vi "Keysight XSAnVMA-Example1.vi"() -> ()   [LabVIEW 2021, in "Keysight XSAnVMA.lvlib"]
doc: "Initializes the driver, reads a few Identity interface properties, and checks the instrument error queue. May include additional instrument specific functionality."
uses:
  <instrlib>/Keysight XSAnVMA/Keysight XSAnVMA.lvlib
  Keysight XSAn/Keysight XSAn.lvlib
panel:
  in  "AttributeValue":dbl=2610000000.0
  in  "DigitalDemodTrace":string="AverageMode"
  out "ValActualSize":i32
  out "Waveform Output":dbl[](array[numeric]) format="%.2p"
  in  "MaxTime":i32=20000 caption="MaxTime (ms)"
  in  "PersonalityName":string="VMA"
  out "Simulation":bool
  out "Identity Properties":string[](array[string])
  out "MESSAGE BOX":string
  in  "option string":string="DriverSetup= Model=, Trace=false, TraceName=c:\\\\temp\\\\traceOut"
  in  "select":bool=TRUE
  in  "Resource string":string="TCPIP0::146.208.245.241::hislip0::INSTR" caption="resource string"
  in  "Simulate":bool=TRUE
  # "Keysight XSAnVMA - Example 1"
  # "SYSTEM_DRIVER_PREFIX"
  # ":"
  # ":"
  # "SYSTEM_DRIVER_REVISION"
  # "SYSTEM_DRIVER_VENDOR"
  # ":"
  # "SPECIFIC_DRIVER_DESCRIPTION"
  # ":"
  # "INSTRUMNET_MODEL"
  # ":"
  # "INSTRUMENT_FIRMWARE_REVISION"
  # ":"
  # "SIMULATE"
  # ":"
  # "© Keysight Technologies 2018 - 2019"
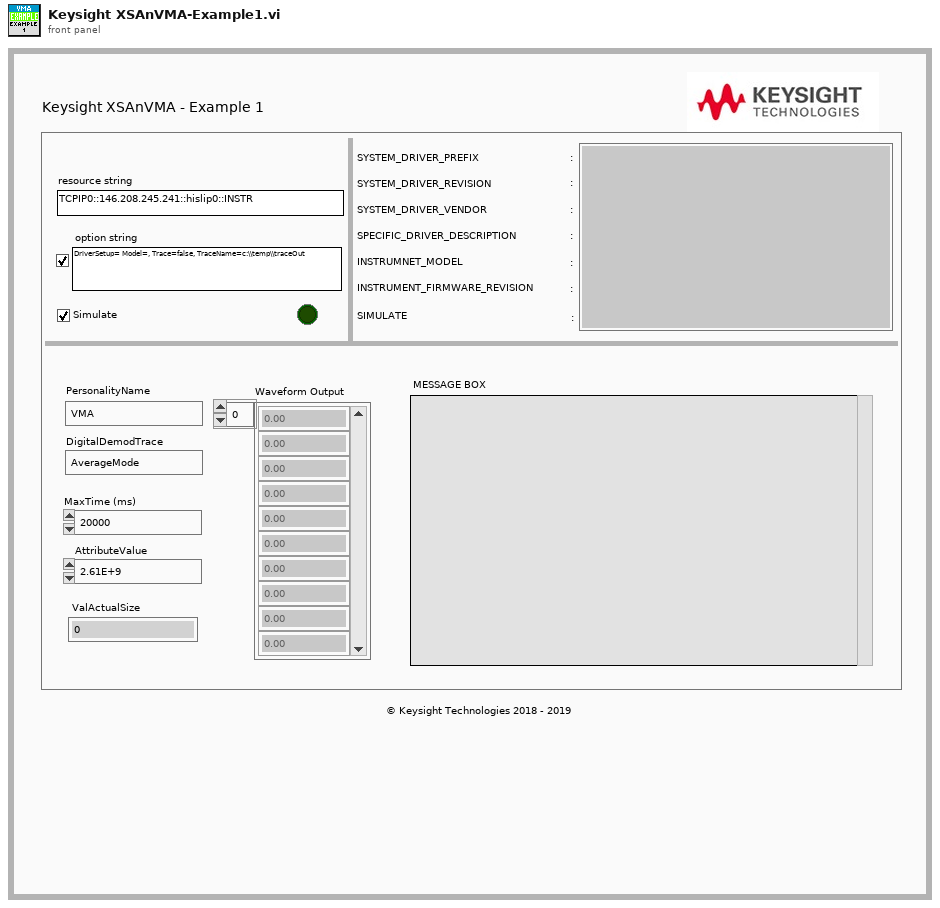
[diagram p1: front panel]
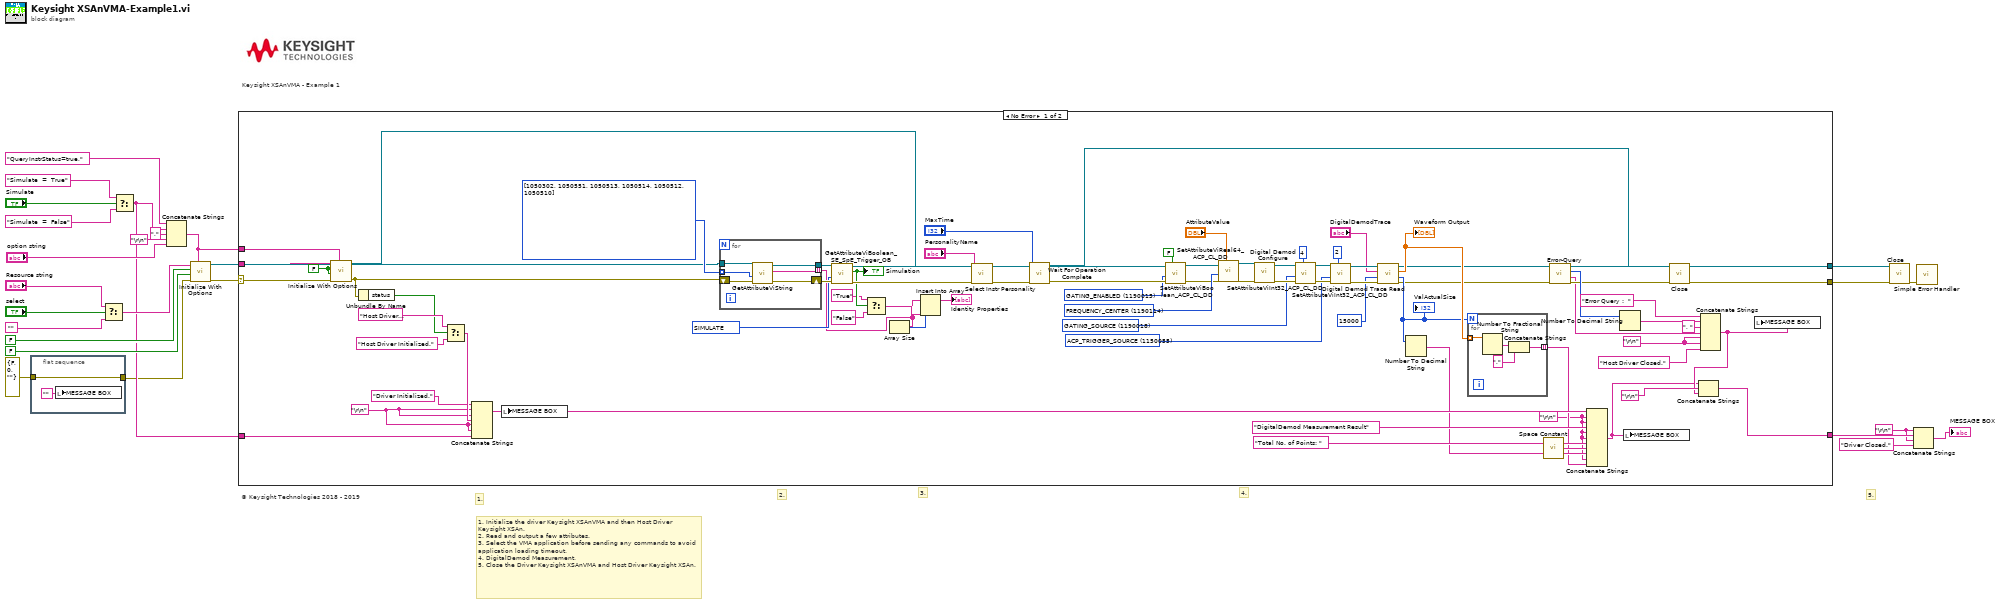
[diagram p0: block diagram]
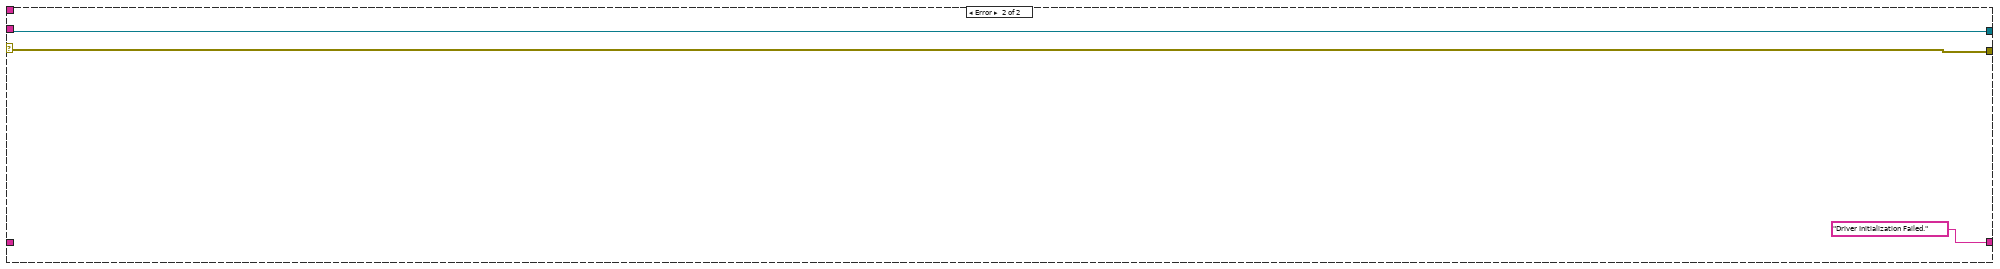
[diagram p2: hidden frame]
diagram:
  w2 = "\r\n"
  # "5."
  # "4."
  # "© Keysight Technologies 2018 - 2019"
  # "3."
  # "2."
  # "Keysight XSAnVMA - Example 1"
  # "1."
  # "1. Initialize the driver Keysight XSAnVMA and then Host Driver Keysight XSAn. \n2. Read and output a few attributes.\n3. Select the VMA application before sending any commands to avoid application loading timeout.\n4. DigitalDemod Measurement.\n5. Close the Driver Keysight XSAnVMA and Host Driver Keysight XSAn."
  n1 = flat-sequence {
    tunnel: errorcluster {"status"=FALSE, "code"=0, "source"=""} ("error in (no error)") -> [w27]
    tunnel: [w27] -> w9
    frame #0 {
      n2 = local write "MESSAGE BOX"("") -> ()
    }
  }
  n3 = Select(t="Resource string", s="select", f="") -> (s? t:f=w12:string)
  n4 = Select(t="Simulate  =  True", s="Simulate", f="Simulate  =  False" ("t")) -> (s? t:f=w11:string)
  n5 = Concatenate Strings("QueryInstrStatus=true," ("t"), w11, "," ("string"), "\r\n", "option string") -> (w13:string)
  n6 = call "Initialize With Options.vi"("option string"=w13, "error in (no error)"=w9, "reset device (Off)"=FALSE ("id query (Off)"), "id query (Off)"=FALSE, "resource string"=w12) -> ("error out"=w3:errorcluster, "instrument handle out"=w14:refnum<k15>)  [unwired: 5 in]
  n7 = case shown="No Error" w3 {
    selector: w3 -> [w41 w119]
    tunnel: w14 -> [w72 w118]
    tunnel: w13 -> [w68 _]
    tunnel: w12 -> [w67 _]
    tunnel: w11 -> [w63 _]
    tunnel: [w36 w119] -> w7
    tunnel: [w43 w118] -> w6
    tunnel: [w33 "Driver Initialization Failed." ("string")] -> w5
    frame No Error {
      w35 = "\r\n"
      w47 = "\r\n"
      w69 = FALSE ("id query (Off)")
      w83 = u32 1150055 items=["ACP_AVERAGE_COUNT"=1150010, "ACP_AVERAGE_MODE"=1150012, "ACP_CARRIER_COUNT"=1150013, "ACP_CARRIER_POWER_REFERENCE_TYPE"=1191309, "ACP_CARRIER_REFERENCE_NUMBER"=1150019, "ACP_DETECTOR_TYPE"=1150003, "ACP_DISPLAY_VIEW_SELECTION"=1191352, "ACP_DISPLAY_WINDOWY_REF_POSITION"=1190656, "ACP_FAST_POWER_IF_GAIN"=1191705, "ACP_FAST_POWER_RBW_MODE"=1191704, "ACP_FREQUENCY_PHASE_NOISE_OPTION_STATE"=1150081, "ACP_MARKER_ACTIVE_MARKER"=1150095, "ACP_MARKER_DELTA_REFERENCE"=1150099, "ACP_MARKER_TRACE"=1150040, "ACP_MARKER_TYPE"=1150102, "ACP_MEASUREMENT_METHOD"=1150006, "ACP_MEASUREMENT_TYPE"=1150007, "ACP_POWER_SPECTRAL_DENSITY_REFERENCE"=1150009, "ACP_SWEEPCOUPLING_BANDWIDTH_SHAPE"=1150001, "ACP_SWEEPCOUPLING_BANDWIDTH_TYPE"=1150002, "ACP_SWEEPCOUPLING_SWEEP_POINTS"=1150025, "ACP_SWEEPCOUPLING_SWEEP_TIME_AUTO_RULES"=1150029, "ACP_TRIGGER_SOURCE"=1150055, "ANALOG_ANTI_ALIASING_FILTER_TYPE"=1191706, "DIGITAL_DEMOD_AVERAGE_COUNT"=1191759, "DIGITAL_DEMOD_AVERAGE_MODE"=1191757, "DIGITAL_DEMOD_CPM_INDEX"=1191642, "DIGITAL_DEMOD_DISPLAY_BITS_FORMAT"=1191625, "DIGITAL_DEMOD_DISPLAY_IDEAL_STATE_SHAPE"=1191615, "DIGITAL_DEMOD_DISPLAY_VIEW_SELECTION"=1191588, "DIGITAL_DEMOD_DISPLAY_WINDOW_TRACE_DATA_FORMAT"=1191665, "DIGITAL_DEMOD_DISPLAY_WINDOW_TRACE_DATA_TYPE"=1191666, "DIGITAL_DEMOD_DISPLAY_WINDOW_X_REF_POSITION"=1191610, "DIGITAL_DEMOD_DISPLAY_WINDOW_X_TIME_UNIT"=1191614, "DIGITAL_DEMOD_DISPLAY_WINDOW_Y_POSITION"=1191592, "DIGITAL_DEMOD_EQUALIZATION_FILTER_LENGTH"=1191634, "DIGITAL_DEMOD_EVM_NORMALIZATION_REFERENCE"=1191667, "DIGITAL_DEMOD_FILTER_REFERENCE"=1191630, "DIGITAL_DEMOD_FILTER_TYPE"=1191627, "DIGITAL_DEMOD_LIMITS_CLOCK_ERROR_UNIT"=1191620, "DIGITAL_DEMOD_LIMITS_FREQUENCY_ERROR_UNIT"=1191621, "DIGITAL_DEMOD_MARKER_ACTIVE_MARKER"=1191593, "DIGITAL_DEMOD_MARKER_DELTA_REFERENCE"=1191596, "DIGITAL_DEMOD_MARKER_FUNCTION"=1191607, "DIGITAL_DEMOD_MARKER_TYPE"=1191601, "DIGITAL_DEMOD_MODULATION_FORMAT"=1191637, "DIGITAL_DEMOD_PHASE_NOISE_OPTIMIZATION"=1191660, "DIGITAL_DEMOD_POINTS_PER_SAMPLE"=1191626, "DIGITAL_DEMOD_SYNC_OFFSET"=1191650, "DIGITAL_DEMOD_TRACE_LIMIT_TYPE"=1191676, "DIGITAL_DEMOD_TRACE_LIMIT_WINDOW_LIMIT"=1191678, "DIGITAL_DEMOD_TRACE_LIMIT_X_REFERENCE"=1191677, "DIGITAL_DEMOD_TRACE_LIMIT_X_UNIT"=1191672, "DIGITAL_DEMOD_TRACE_LIMIT_Y_UNIT"=1191761, "DIGITAL_DEMOD_TRIGGER_SOURCE"=1191613, "GATING_DELAY_COMPENSATION"=1150141, "GATING_SOURCE"=1190018, "GATING_TYPE"=1190019, "INPUT_IQ_FEED_TYPE"=1190844, "INPUT_IQ_I_COUPLING"=1191695, "INPUT_IQ_I_IMPEDANCE"=1191701, "INPUT_IQ_IMPEDANCE"=1191699, "INPUT_IQ_Q_COUPLING"=1191696, "INPUT_IQ_Q_IMPEDANCE"=1191702, "INPUT_RF_PRE_AMPLIFIER_BAND"=1190118, "LEVEL_ATTENUATION_OPTIMIZE"=1190119, "LEVEL_ATTENUATION_STEP_INCREMENT"=1190120] ("AttributeID")
      w87 = u32 1190018 items=["ACP_AVERAGE_COUNT"=1150010, "ACP_AVERAGE_MODE"=1150012, "ACP_CARRIER_COUNT"=1150013, "ACP_CARRIER_POWER_REFERENCE_TYPE"=1191309, "ACP_CARRIER_REFERENCE_NUMBER"=1150019, "ACP_DETECTOR_TYPE"=1150003, "ACP_DISPLAY_VIEW_SELECTION"=1191352, "ACP_DISPLAY_WINDOWY_REF_POSITION"=1190656, "ACP_FAST_POWER_IF_GAIN"=1191705, "ACP_FAST_POWER_RBW_MODE"=1191704, "ACP_FREQUENCY_PHASE_NOISE_OPTION_STATE"=1150081, "ACP_MARKER_ACTIVE_MARKER"=1150095, "ACP_MARKER_DELTA_REFERENCE"=1150099, "ACP_MARKER_TRACE"=1150040, "ACP_MARKER_TYPE"=1150102, "ACP_MEASUREMENT_METHOD"=1150006, "ACP_MEASUREMENT_TYPE"=1150007, "ACP_POWER_SPECTRAL_DENSITY_REFERENCE"=1150009, "ACP_SWEEPCOUPLING_BANDWIDTH_SHAPE"=1150001, "ACP_SWEEPCOUPLING_BANDWIDTH_TYPE"=1150002, "ACP_SWEEPCOUPLING_SWEEP_POINTS"=1150025, "ACP_SWEEPCOUPLING_SWEEP_TIME_AUTO_RULES"=1150029, "ACP_TRIGGER_SOURCE"=1150055, "ANALOG_ANTI_ALIASING_FILTER_TYPE"=1191706, "DIGITAL_DEMOD_AVERAGE_COUNT"=1191759, "DIGITAL_DEMOD_AVERAGE_MODE"=1191757, "DIGITAL_DEMOD_CPM_INDEX"=1191642, "DIGITAL_DEMOD_DISPLAY_BITS_FORMAT"=1191625, "DIGITAL_DEMOD_DISPLAY_IDEAL_STATE_SHAPE"=1191615, "DIGITAL_DEMOD_DISPLAY_VIEW_SELECTION"=1191588, "DIGITAL_DEMOD_DISPLAY_WINDOW_TRACE_DATA_FORMAT"=1191665, "DIGITAL_DEMOD_DISPLAY_WINDOW_TRACE_DATA_TYPE"=1191666, "DIGITAL_DEMOD_DISPLAY_WINDOW_X_REF_POSITION"=1191610, "DIGITAL_DEMOD_DISPLAY_WINDOW_X_TIME_UNIT"=1191614, "DIGITAL_DEMOD_DISPLAY_WINDOW_Y_POSITION"=1191592, "DIGITAL_DEMOD_EQUALIZATION_FILTER_LENGTH"=1191634, "DIGITAL_DEMOD_EVM_NORMALIZATION_REFERENCE"=1191667, "DIGITAL_DEMOD_FILTER_REFERENCE"=1191630, "DIGITAL_DEMOD_FILTER_TYPE"=1191627, "DIGITAL_DEMOD_LIMITS_CLOCK_ERROR_UNIT"=1191620, "DIGITAL_DEMOD_LIMITS_FREQUENCY_ERROR_UNIT"=1191621, "DIGITAL_DEMOD_MARKER_ACTIVE_MARKER"=1191593, "DIGITAL_DEMOD_MARKER_DELTA_REFERENCE"=1191596, "DIGITAL_DEMOD_MARKER_FUNCTION"=1191607, "DIGITAL_DEMOD_MARKER_TYPE"=1191601, "DIGITAL_DEMOD_MODULATION_FORMAT"=1191637, "DIGITAL_DEMOD_PHASE_NOISE_OPTIMIZATION"=1191660, "DIGITAL_DEMOD_POINTS_PER_SAMPLE"=1191626, "DIGITAL_DEMOD_SYNC_OFFSET"=1191650, "DIGITAL_DEMOD_TRACE_LIMIT_TYPE"=1191676, "DIGITAL_DEMOD_TRACE_LIMIT_WINDOW_LIMIT"=1191678, "DIGITAL_DEMOD_TRACE_LIMIT_X_REFERENCE"=1191677, "DIGITAL_DEMOD_TRACE_LIMIT_X_UNIT"=1191672, "DIGITAL_DEMOD_TRACE_LIMIT_Y_UNIT"=1191761, "DIGITAL_DEMOD_TRIGGER_SOURCE"=1191613, "GATING_DELAY_COMPENSATION"=1150141, "GATING_SOURCE"=1190018, "GATING_TYPE"=1190019, "INPUT_IQ_FEED_TYPE"=1190844, "INPUT_IQ_I_COUPLING"=1191695, "INPUT_IQ_I_IMPEDANCE"=1191701, "INPUT_IQ_IMPEDANCE"=1191699, "INPUT_IQ_Q_COUPLING"=1191696, "INPUT_IQ_Q_IMPEDANCE"=1191702, "INPUT_RF_PRE_AMPLIFIER_BAND"=1190118, "LEVEL_ATTENUATION_OPTIMIZE"=1190119, "LEVEL_ATTENUATION_STEP_INCREMENT"=1190120] ("AttributeID")
      w94 = u32 1190114 items=["ACP_CARRIER_CPSD"=1150014, "ACP_CARRIER_REFERENCE_FREQUENCY"=1150015, "ACP_CARRIER_REFERENCE_LEVEL"=1150017, "ACP_DISPLAY_WINDOWY_REFERENCE"=1150091, "ACP_DISPLAY_WINDOWY_SCALE"=1150092, "ACP_FREQUENCY_SPAN"=1150094, "ACP_INTEGRATION_BANDWIDTH"=1191694, "ACP_MARKER_POSITION"=1150101, "ACP_MARKER_TRACE_POINTS_POSITION"=1190657, "ACP_OFFSET_FILTER_ALPHA"=1150103, "ACP_SWEEPCOUPLING_RESOLUTION_BANDWIDTH"=1150023, "ACP_SWEEPCOUPLING_SWEEP_TIME"=1150027, "ACP_SWEEPCOUPLING_VIDEO_BANDWIDTH"=1150030, "DIGITAL_DEMOD_ADJUST_CLOCK"=1191641, "DIGITAL_DEMOD_APSK_RING2_RATIO"=1191631, "DIGITAL_DEMOD_APSK_RING3_RATIO"=1191632, "DIGITAL_DEMOD_DISPLAY_IDEAL_STATE_SIZE"=1191616, "DIGITAL_DEMOD_DISPLAY_WINDOW_X_REFERENCE"=1191609, "DIGITAL_DEMOD_DISPLAY_WINDOW_X_WIDTH"=1191658, "DIGITAL_DEMOD_DISPLAY_WINDOW_Y_REFERENCE"=1191591, "DIGITAL_DEMOD_DISPLAY_WINDOW_Y_SCALE"=1191590, "DIGITAL_DEMOD_EQUALIZATION_CONVERGENCE"=1191636, "DIGITAL_DEMOD_FILTER_ALPHA"=1191628, "DIGITAL_DEMOD_FILTER_BETA"=1191629, "DIGITAL_DEMOD_FSK_DEVIATION_REFERENCE"=1191638, "DIGITAL_DEMOD_FSK_TX_FREQUENCY_OFFSET"=1191640, "DIGITAL_DEMOD_IQ_ROTATION"=1191664, "DIGITAL_DEMOD_LIMITS_CLOCK_ERROR_IN_HERTZ"=1191619, "DIGITAL_DEMOD_LIMITS_CLOCK_ERROR_INPPM"=1191622, "DIGITAL_DEMOD_LIMITS_DEVIATION_ACCURACY"=1191647, "DIGITAL_DEMOD_LIMITS_FREQUENCY_ERROR_IN_HERTZ"=1191618, "DIGITAL_DEMOD_LIMITS_FREQUENCY_ERROR_INPPM"=1191623, "DIGITAL_DEMOD_LIMITS_POWER_LIMIT"=1191624, "DIGITAL_DEMOD_LIMITS_RMS_FSK_ERROR"=1191646, "DIGITAL_DEMOD_LIMITS_RMS_OFFSETEVM"=1191648, "DIGITAL_DEMOD_MARKER_FUNCTION_BAND_LEFT"=1191602, "DIGITAL_DEMOD_MARKER_FUNCTION_BAND_RIGHT"=1191603, "DIGITAL_DEMOD_MARKER_FUNCTION_BAND_SPAN"=1191604, "DIGITAL_DEMOD_MARKER_POSITION"=1191599, "DIGITAL_DEMOD_MARKER_WINDOW_TRACE"=1191681, "DIGITAL_DEMOD_MARKER_Y_IMAGINARY"=1191682, "DIGITAL_DEMOD_MULTI_CARRIER_FILTER_BANDWIDTH"=1191680, "DIGITAL_DEMOD_SAMPLE_RATE"=1191617, "DIGITAL_DEMOD_SWEEP_COUPLING_RESOLUTION_BANDWIDTH"=1191762, "DIGITAL_DEMOD_SYMBOL_INTERVAL"=1191659, "DIGITAL_DEMOD_SYNC_BURST_SEARCH_THRESHOLD"=1191652, "DIGITAL_DEMOD_SYNC_SEARCH_LENGTH"=1191653, "DIGITAL_DEMOD_TRACE_LIMIT_MARGIN"=1191674, "DIGITAL_DEMOD_TRACE_LIMIT_X_OFFSET"=1191673, "DIGITAL_DEMOD_TRACE_LIMIT_Y_OFFSET"=1191760, "FREQUENCY_CENTER"=1190114, "FREQUENCY_CENTER_STEP"=1150133, "GATING_DELAY"=1190014, "GATING_HOLD_OFF_TIME"=1150142, "GATING_LENGTH"=1190016, "GATING_VIEW_START_TIME"=1191460, "GATING_VIEW_SWEEP_TIME"=1190021, "INPUT_IQ_CENTER_FREQUENCY"=1191715, "INPUT_IQ_I_ATTENUATION"=1190851, "INPUT_IQ_I_ATTENUATION_RATIO"=1190853, "INPUT_IQ_I_EXTERNAL_GAIN"=1190840, "INPUT_IQ_I_OFFSET"=1191697, "INPUT_IQ_I_SKEW_FACTOR"=1190843, "INPUT_IQ_Q_ATTENUATION_RATIO"=1190854, "INPUT_IQ_Q_ATTENUATION"=1190852, "INPUT_IQ_Q_EXTERNAL_GAIN"=1190841, "INPUT_IQ_Q_OFFSET"=1191698, "INPUT_IQ_Q_SKEW_FACTOR"=1190842, "INPUT_IQ_REFERENCE_IMPEDANCE"=1191700, "INPUT_RF_BASE_STATION_GAIN"=1190115, "INPUT_RF_MOBILE_STATION_GAIN"=1190116, "LEVEL_ATTENUATION"=1190002, "LEVEL_ELECTRONIC_ATTENUATION"=1190121] ("AttributeID")
      w96 = u32 1190015 items=["ACP_AVERAGE_ENABLED"=1150011, "ACP_CARRIER_REFERENCE_FREQUENCY_AUTO_ENABLED"=1150016, "ACP_CARRIER_REFERENCE_LEVEL_AUTO_ENABLED"=1150018, "ACP_CARRIER_REFERENCE_NUMBER_AUTO_ENABLED"=1150020, "ACP_DETECTOR_AUTO_ENABLED"=1150058, "ACP_DISPLAY_BAR_GRAPH_ENABLED"=1150089, "ACP_DISPLAY_WINDOWY_AUTO_SCALE_ENABLED"=1150093, "ACP_FREQUENCY_PHASE_NOISE_OPTION_AUTO_ENABLED"=1150072, "ACP_LIMIT_TEST_ENABLED"=1150005, "ACP_LIMIT_TEST_FAIL_STATE"=1150004, "ACP_MARKER_COUPLE_ENABLED"=1150098, "ACP_MARKER_ENABLED"=1150100, "ACP_NOISE_CORRECTION_ENABLED"=1150008, "ACP_OFFSET_FILTER_ENABLED"=1150104, "ACP_SWEEPCOUPLING_RESOLUTION_BANDWIDTH_AUTO_ENABLED"=1150024, "ACP_SWEEPCOUPLING_SWEEP_TIME_AUTO_ENABLED"=1150028, "ACP_SWEEPCOUPLING_VIDEO_BANDWIDTH_AUTO_ENABLED"=1150033, "ANALOG_ANTI_ALIASING_FILTER_AUTO_ENABLED"=1191707, "AUTO_SCALE_ENABLED"=1191693, "CONTINUOUS_PEAK_SEARCH_ENABLED"=1191709, "DIGITAL_DEMOD_AVERAGE_ENABLED"=1191758, "DIGITAL_DEMOD_CPM_AUTO_ENABLED"=1191643, "DIGITAL_DEMOD_DISPLAY_WINDOW_X_AUTO_SCALE_ENABLED"=1191608, "DIGITAL_DEMOD_EQUALIZATION_ENABLED"=1191633, "DIGITAL_DEMOD_EQUALIZATION_HOLD_ENABLED"=1191635, "DIGITAL_DEMOD_FSK_DEVIATION_REFERENCE_AUTO_ENABLED"=1191639, "DIGITAL_DEMOD_IF_GAIN"=1191656, "DIGITAL_DEMOD_IF_GAIN_AUTO_ENABLED"=1191657, "DIGITAL_DEMOD_IQ_NORMALIZATION_ENABLED"=1191645, "DIGITAL_DEMOD_IQ_OFFSET_COMPENSATION_ENABLED"=1191663, "DIGITAL_DEMOD_LIMIT_TEST_ENABLED"=1191612, "DIGITAL_DEMOD_LOW_SNR_ENHANCEMENT_ENABLED"=1191649, "DIGITAL_DEMOD_MARKER_COUPLE_ENABLED"=1191606, "DIGITAL_DEMOD_MARKER_ENABLED"=1191597, "DIGITAL_DEMOD_MULTI_CARRIER_FILTER_ENABLED"=1191679, "DIGITAL_DEMOD_QUAD_SKEW_COUPLING_ENABLED"=1191644, "DIGITAL_DEMOD_SYNC_BURST_SEARCH_ENABLED"=1191654, "DIGITAL_DEMOD_SYNC_SEARCH_ENABLED"=1191651, "DIGITAL_DEMOD_TRACE_LIMIT_DISPLAY_ENABLED"=1191669, "DIGITAL_DEMOD_TRACE_LIMIT_MARGIN_AUTO_ENABLED"=1191675, "FREQUENCY_CENTER_STEP_AUTO_ENABLED"=1150134, "GATING_ENABLED"=1190015, "GATING_HOLD_OFF_TIME_AUTO_ENABLED"=1150143, "GATING_VIEW"=1190020, "INPUT_IQ_I_DIFFERENTIAL_ENABLED"=1191713, "INPUT_IQ_MIRROR_ENABLED"=1191712, "INPUT_IQ_Q_DIFFERENTIAL_ENABLED"=1191714, "INPUT_RF_PRE_AMP_ENABLED"=1190117, "LEVEL_ELECTRONIC_ATTENUATION_STATE_ENABLED"=1190122, "SIMULATE"=1050005] ("AttributeID")
      w106 = u32[] [1050302, 1050551, 1050513, 1050514, 1050512, 1050510] items=["ACP_DISPLAY_TEXT"=1150090, "CHANNELPOWER_DISPLAY_TITLE"=1190233, "DIGITAL_DEMOD_DISPLAY_TEXT"=1191586, "DIGITAL_DEMOD_SYNC_PATTERN"=1191655, "DIGITAL_DEMOD_TRACE_LIMIT_COMMENT"=1191671, "DIGITAL_DEMOD_TRACE_LIMIT_DESCRIPTION"=1191670, "DRIVER_SETUP"=1050007, "INSTRUMENT_FIRMWARE_REVISION"=1050510, "INSTRUMENT_MANUFACTURER"=1050511, "INSTRUMENT_MODEL"=1050512, "IO_RESOURCE_DESCRIPTOR"=1050304, "LOGICAL_NAME"=1050305, "MONITOR_DISPLAY_TITLE"=1190351, "OCCUPIED_BANDWIDTH_DISPLAY_TEXT"=1190390, "POWER_STATISTICS_DISPLAY_TEXT"=1190433, "SEMASK_DISPLAY_TEXT"=1190491, "SPECIFIC_DRIVER_DESCRIPTION"=1050514, "SPECIFIC_DRIVER_PREFIX "=1050302, "SPECIFIC_DRIVER_REVISION"=1050551, "SPECIFIC_DRIVER_VENDOR"=1050513, "SPURIOUS_EMISSIONS_DISPLAY_TEXT"=1190519, "SUPPORTED_INSTRUMENT_MODELS"=1050327, "WAVEFORM_DISPLAY_TITLE"=1190543]
      w57 = "\r\n"
      w103 = u32 1050005 items=["ANALYZER_BIT_RECOVERY_MODE_ENABLED"=1150360, "CDR_AUTO_ENABLED"=1150344, "CDR_ENABLED"=1150020, "CDR_HIGH_TRANSITION_DENSITY"=1150345, "CLOCK_OUTPUT_ENABLED"=1150261, "CLOCK_OUTPUT_HIGH_FREQUENCY_JITTER_BOUNDED_UNCORRELATED_JITTER_ENABLED"=1150302, "CLOCK_OUTPUT_HIGH_FREQUENCY_JITTER_EXTERNAL_JITTER_SOURCE_ENABLED"=1150266, "CLOCK_OUTPUT_HIGH_FREQUENCY_JITTER_PERIODIC_JITTER_SOURCE1_ENABLED"=1150267, "CLOCK_OUTPUT_HIGH_FREQUENCY_JITTER_PERIODIC_JITTER_SOURCE2_ENABLED"=1150268, "CLOCK_OUTPUT_HIGH_FREQUENCY_JITTER_RANDOM_JITTER_SOURCE_ENABLED"=1150269, "CLOCK_OUTPUT_HIGH_FREQUENCY_JITTER_SPECTRAL_JITTER_SOURCE_ENABLED"=1150270, "CLOCK_OUTPUT_LOW_FREQUENCY_JITTER_PERIODIC_ENABLED"=1150276, "CLOCK_OUTPUT_LOW_FREQUENCY_JITTER_RESIDUAL_SPREAD_SPECTRUM_CLOCKING_ENABLED"=1150279, "CLOCK_SYMBOL_RATE_TRACKING_ENABLED"=1150372, "COMMON_MODE_ENABLED"=1150097, "CONTROL_OUT_A_ENABLED"=1150243, "DATA_OUTPUT_TIMING_HIGH_JITTER_INJECTION_MODE_ENABLED"=1150129, "DATAOUT_AMPLIFIER_ENABLED"=1150060, "DATAOUT_AMPLIFIER_F2_JITTER_ENABLED"=1150375, "DATAOUT_AMPLIFIER_RANGE_AUTO_ENABLED"=1150056, "DATAOUT_LINE_CODING_PRE_CODER_ENABLED"=1150367, "DE_EMBEDDING_CABLE_COMPENSATION_STATE_ENABLED"=1150346, "DE_EMBEDDING_S_PARAMETER_ENABLED"=1150350, "DEEMPHASIS_AUTO_ADJUST_MAIN_CURSOR_ENABLED"=1150362, "DIFFERENTIAL_MODE_ENABLED"=1150100, "EMBEDDING_S_PARAMETER_ENABLED"=1150336, "ENABLED"=1150396, "ERROR_INSERTION_ENABLED"=1150068, "ERROR_RATIO_ACQUISITION_STATUS_IS_RUNNING"=1150404, "ERROR_RATIO_SHOW_GRAPH_LEGEND_ENABLED"=1150151, "EYE_DIAGRAM_ACQUISITION_STATUS_IS_RUNNING"=1150408, "EYE_DIAGRAM_DISPLAY_CONTOUR_LEGEND"=1150328, "EYE_DIAGRAM_DISPLAY_CONTOUR_LINES"=1150327, "EYE_DIAGRAM_DISPLAY_WAVEFORM_ENABLED"=1150329, "EYE_DIAGRAM_DISPLAY_WAVEFORM_SMOOTHING_MODE_ENABLED"=1150330, "HIGH_FREQUENCY_JITTER_BOUNDED_UNCORRELATED_ENABLED"=1150074, "HIGH_FREQUENCY_JITTER_EXTERNAL_STATE"=1150072, "HIGH_FREQUENCY_JITTER_RANDOM_ENABLED"=1150091, "HIGH_FREQUENCY_JITTER_SPECTRAL_ENABLED"=1150089, "HIGH_FREQUENCY_JITTER_SPECTRAL_LOW_PASS_FILTER_ENABLED"=1150088, "INTER_SYMBOL_INTERFERENCE_ENABLED"=1150110, "JITTER_SWEEP_ENABLED"=1150117, "JITTER_TOLERANCE_ACQUISITION_STATUS_IS_RUNNING"=1150410, "JITTER_TOLERANCE_GRAPH_COMPLIANCE_LIMITS_ENABLED"=1150158, "JITTER_TOLERANCE_GRAPH_TEMPLATE_LIMITS_ENABLED"=1150159, "JITTER_TOLERANCE_GRAPH_TEMPLATE_POINTS_ENABLED"=1150160, "JITTER_TOLERANCE_HISTORY_ENABLED"=1150400, "JITTER_TOLERANCE_MEASUREMENT_SETUP_CDR_LOOP_BANDWIDTH_AUTO_ENABLED"=1150364, "JITTER_TOLERANCE_MEASUREMENT_SETUP_TEMPLATE_POINTS_ENABLED"=1150171, "LOW_FREQUENCY_JITTER_PERIODIC_ENABLED"=1150137, "LOW_FREQUENCY_JITTER_RESIDUAL_SPREAD_SPECTRUM_CLOCKING_ENABLED"=1150138, "MODULE_GLOBAL_JITTER_ENABLED"=1150304, "MODULE_GLOBAL_OUTPUT_ENABLED"=1150305, "OUTPUT_LEVEL_ACQUISITION_ERROR_BIT_ENABLED"=1150176, "OUTPUT_LEVEL_ACQUISITION_STATUS_IS_RUNNING"=1150413, "OUTPUT_LEVEL_DISPLAY_GRAPH_LEGEND_ENABLED"=1150183, "OUTPUT_LEVEL_DISPLAY_MEASUREMENTS_POINT_ENABLED"=1150184, "OUTPUT_LEVEL_HISTORY_ENABLED"=1150399, "OUTPUT_TIMING_ACQUISITION_ERROR_BIT_ENABLED"=1150199, "OUTPUT_TIMING_ACQUISITION_OPTIMIZATION"=1150203, "OUTPUT_TIMING_ACQUISITION_STATUS_IS_RUNNING"=1150416, "OUTPUT_TIMING_DISPLAY_GRAPH_LEGEND_ENABLED"=1150211, "OUTPUT_TIMING_DISPLAY_MEASUREMENT_POINTS_ENABLED"=1150212, "OUTPUT_TIMING_HISTORY_ENABLED"=1150398, "PATTERN_CAPTURE_ACQUISITION_STATUS_IS_RUNNING"=1150419, "QUERY_INSTRUMENT_STATUS"=1050003, "SIMULATE"=1050005, "SPREAD_SPECTRUM_CLOCKING_ENABLED"=1150287, "SPREAD_SPECTRUM_CLOCKING_GLOBAL_MODE_ENABLED"=1150357, "SYSTEM_OUT_A_AMPLIFIER_ENABLED"=1150234, "SYSTEM_OUT_B_AMPLIFIER_ENABLED"=1150229, "TRIGGER_AMPLIFIER_ENABLED"=1150223] ("Attribute ID")
      n8 = call "Initialize With Options.vi"("option string"=w68, "error in (no error)"=w41, "reset device (Off)"=w69, "id query (Off)"=w69, "resource string"=w67) -> ("error out"=w62:errorcluster, "instrument handle out"=w70:refnum<k15>)  [unwired: 5 in]
      n9 = Unbundle By Name(w62) -> ("status"=w59:bool)
      n10 = Select(t="Host Driver Initialization Failed." ("string"), s=w59, f="Host Driver Initialized." ("string")) -> (s? t:f=w58:string)
      n11 = Concatenate Strings("Driver Initialized." ("string"), w57, w57, w58, w57, w57, w63) -> (w56:string)
      n12 = local write "MESSAGE BOX"(w56) -> ()
      n13 = for {
        tunnel: w106 -> [w111] mode=indexing
        tunnel: [w112] -> w73 mode=indexing
        shift-right: [w113] -> w104
        shift-left: w62 -> [w115]
        tunnel: w72 -> [w116]
        tunnel: [w114] -> w105
        n14 = call <instrlib>:"GetAttributeViString.vi"("error in (no error)"=w115, "AttributeID"=w111, "instrument handle"=w116) -> ("error out"=w113:errorcluster, "AttributeValue"=w112:string, "instrument handle out"=w114:refnum<k15>)  [unwired: 6 in]
      }
      n15 = call <instrlib>:"GetAttributeViBoolean_SE_SpE_Trigger_OB.vi"("error in (no error)"=w104, "AttributeID"=w103, "instrument handle"=w105) -> ("error out"=w102:errorcluster, "AttributeValue"=w78:bool, "instrument handle out"=w65:refnum<k15>)  [unwired: 6 in]
      "Simulation" <- w78
      n16 = Select(t="True" ("Module 2"), s=w78, f="False" ("Module 2")) -> (s? t:f=w75:string)
      n17 = Array Size(array=w73) -> (size(s)=w74:i32)
      n18 = Insert Into Array(array=w73, index=w74, new element=w75) -> (→"Identity Properties":string[])
      n19 = call <instrlib>:"Select Instr Personality.vi"("error in (no error)"=w102, "PersonalityName"="PersonalityName", "instrument handle"=w70) -> ("error out"=w98:errorcluster, "instrument handle out"=w99:refnum<k15>)  [unwired: 7 in]
      n20 = call <instrlib>:"Wait For Operation Complete.vi"("error in (no error)"=w98, "MaxTime"="MaxTime", "instrument handle"=w99) -> ("error out"=w97:errorcluster, "instrument handle out"=w64:refnum<k15>)  [unwired: 7 in]
      n21 = call <instrlib>:"SetAttributeViBoolean_ACP_CL_DD.vi"("AttributeValue (Off)"=FALSE, "error in (no error)"=w97, "AttributeID"=w96, "instrument handle"=w65) -> ("error out"=w90:errorcluster, "instrument handle out"=w95:refnum<k15>)  [unwired: 6 in]
      n22 = call <instrlib>:"SetAttributeViReal64_ACP_CL_DD.vi"("AttributeValue"="AttributeValue", "error in (no error)"=w90, "AttributeID"=w94, "instrument handle"=w95) -> ("error out"=w92:errorcluster, "instrument handle out"=w91:refnum<k15>)  [unwired: 6 in]
      n23 = call <instrlib>:"Digital Demod Configure.vi"("error in (no error)"=w92, "instrument handle"=w91) -> ("error out"=w88:errorcluster, "instrument handle out"=w89:refnum<k15>)  [unwired: 8 in]
      n24 = call <instrlib>:"SetAttributeViInt32_ACP_CL_DD.vi"("AttributeValue"=4, "error in (no error)"=w88, "AttributeID"=w87, "instrument handle"=w89) -> ("error out"=w85:errorcluster, "instrument handle out"=w84:refnum<k15>)  [unwired: 6 in]
      n25 = call <instrlib>:"SetAttributeViInt32_ACP_CL_DD.vi"("AttributeValue"=2, "error in (no error)"=w85, "AttributeID"=w83, "instrument handle"=w84) -> ("error out"=w80:errorcluster, "instrument handle out"=w81:refnum<k15>)  [unwired: 6 in]
      n26 = call <instrlib>:"Digital Demod Trace Read.vi"("error in (no error)"=w80, "MaxTimeMilliseconds"=15000, "DigitalDemodTrace"="DigitalDemodTrace", "instrument handle"=w81) -> ("error out"=w38:errorcluster, "ValActualSize"=w48:i32, "Val"=w50:dbl[], "instrument handle out"=w44:refnum<k15>)  [unwired: 4 in]
      "Waveform Output" <- w50
      "ValActualSize" <- w48
      n27 = Number To Decimal String(number=w48) -> (decimal integer string=w51:string)  [unwired: 1 in]
      n28 = for {
        N: w48 -> [_]
        tunnel: w50 -> [w110] mode=indexing
        tunnel: [w107] -> w49 mode=indexing
        n29 = Number To Fractional String(number=w110) -> (F-format string=w109:string)  [unwired: 3 in]
        n30 = Concatenate Strings(w109, "," ("string")) -> (w107:string)
      }
      n31 = call <vilib>:"Space Constant.vi"() -> ("String"=w52:string)
      n32 = call "Error-Query.vi"("error in (no error)"=w38, "instrument handle"=w44) -> ("error out"=w37:errorcluster, "error message"=w30:string, "error code"=w42:i32, "instrument handle out"=w43:refnum<k15>)  [unwired: 6 in]
      n33 = Concatenate Strings(w56, w47, w47, "DigitalDemod Measurement Result" ("concatenated string"), w47, w47, "Total No. of Points: " ("string"), w52, w51, w47, w49) -> (w32:string)
      n34 = Number To Decimal String(number=w42) -> (decimal integer string=w45:string)  [unwired: 1 in]
      n35 = local write "MESSAGE BOX"(w32) -> ()
      n36 = call "Close.vi"("error in (no error)"=w37, "instrument handle"=w64) -> ("error out"=w36:errorcluster)  [unwired: 9 in]
      n37 = Concatenate Strings("Error Query :  " ("string"), w45, ", " ("string"), w30, w35, w35, "Host Driver Closed." ("string")) -> (w34:string)
      n38 = Concatenate Strings(w32, "\r\n", w34) -> (w33:string)
      n39 = local write "MESSAGE BOX"(w34) -> ()
    }
    frame Error {
    }
  }
  n40 = call "Close.vi"("error in (no error)"=w7, "instrument handle"=w6) -> ("error out"=w8:errorcluster)  [unwired: 9 in]
  n41 = Concatenate Strings(w2, w5, w2, "Driver Closed." ("string")) -> (→"MESSAGE BOX":string)
  n42 = call <vilib>:"Simple Error Handler.vi"("error in (no error)"=w8) -> ()  [unwired: 4 in, 5 out]
